vi "Get Config Hash.vi"(8 "error in (no error)":errorcluster, 11 "Node Config in":refnum<class "Node Config.lvclass">) -> (0 "error out":errorcluster, 2 "Config Hash":string, 3 "Node Config out":refnum<class "Node Config.lvclass">)   [LabVIEW 2020, in "VectoConfig.lvlib" / "Node Config.lvclass"]
uses:
  Node Config.lvclass
  Node Config.lvclass/Node Config.ctl
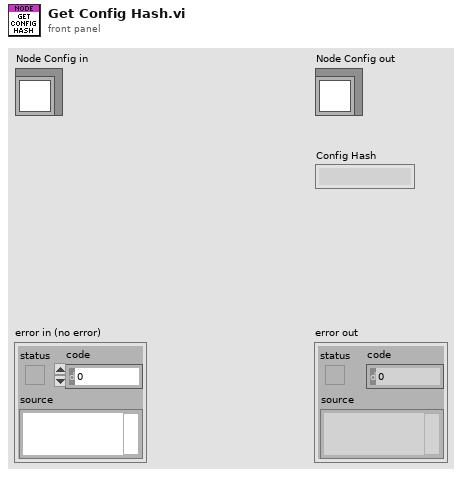
[diagram p1: front panel]
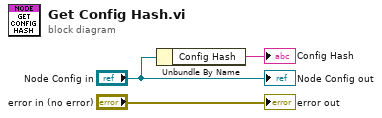
[diagram p0: block diagram]
diagram:
  n1 = Unbundle By Name("Node Config in") -> ("Config Hash"=→"Config Hash":string)
  "error out" <- "error in (no error)"
  "Node Config out" <- "Node Config in"
